vi "Create Properties.vi"(5 "Properties in":refnum<class "Properties.lvclass">, 6 "timestamp (now)":timestamp, 7 "label":string, 8 "call-chain":string[](array[string]), 9 "self-id":string, 10 "owner-id":string, 11 "Test Manager":refnum<class "Basic Test Manager.lvclass">) -> (3 "Properties out":refnum<class "Properties.lvclass">)   [LabVIEW 2013, in "Caraya.lvlib" / "Properties.lvclass"]
uses:
  Properties.lvclass
  Basic Test Manager/Basic Test Manager.lvclass
  Properties.lvclass/Properties.ctl
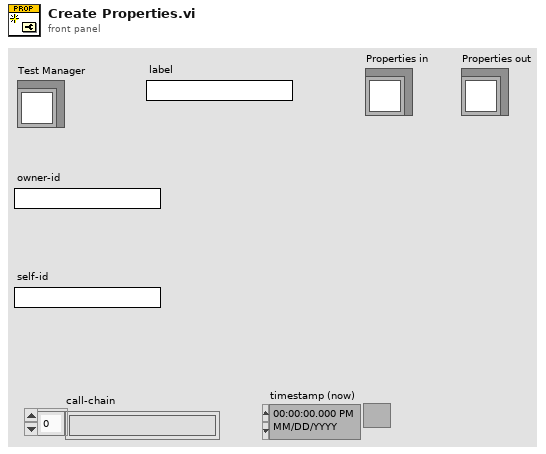
[diagram p1: front panel]
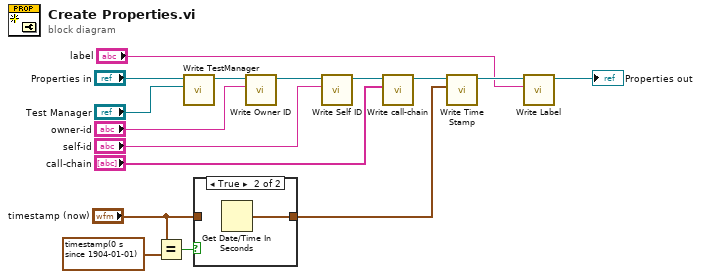
[diagram p0: block diagram]
diagram:
  n1 = Equal?(x="timestamp (now)", y=timestamp(0 s since 1904-01-01)) -> (x = y?=w5:bool)
  n2 = call "Write TestManager.vi"("Test Manager"="Test Manager", "Properties in"="Properties in") -> ("Properties out"=w15:refnum<class "Properties.lvclass">)  [unwired: 9 in]
  n3 = case shown="True" w5 {
    tunnel: [w17 w18] -> w16
    tunnel: "timestamp (now)" -> [w17 _]
    frame False {
    }
    frame True {
      n4 = Get Date/Time In Seconds() -> (seconds since 1Jan1904=w18:timestamp)
    }
  }
  n5 = call "Write Owner ID.vi"("owner-id"="owner-id", "Properties in"=w15) -> ("Properties out"=w14:refnum<class "Properties.lvclass">)  [unwired: 9 in]
  n6 = call "Write Self ID.vi"("self-id"="self-id", "Properties in"=w14) -> ("Properties out"=w13:refnum<class "Properties.lvclass">)  [unwired: 9 in]
  n7 = call "Write call-chain.vi"("call-chain"="call-chain", "Properties in"=w13) -> ("Properties out"=w12:refnum<class "Properties.lvclass">)  [unwired: 9 in]
  n8 = call "Write Time Stamp.vi"("timestamp"=w16, "Properties in"=w12) -> ("Properties out"=w3:refnum<class "Properties.lvclass">)  [unwired: 9 in]
  n9 = call "Write Label.vi"("Label"="label", "Properties in"=w3) -> ("Properties out"=→"Properties out":refnum<class "Properties.lvclass">)  [unwired: 9 in]
